vi "log_message.vi"(6 "timestamp":timestamp, 7 "context":string, 8 "error in (no error)":errorcluster, 9 "level":T1=400 items=["OFF"=0, "FATAL"=100, "ERROR"=200, "WARN"=300, "INFO"=400, "DEBUG"=500, "TRACE"=600, "ALL"=65535], 10 "message":string, 11 "Log Service in":refnum<class "Log Service.lvclass">) -> (0 "error out":errorcluster, 3 "Log Service out":refnum<class "Log Service.lvclass">)   [LabVIEW 2019, in "LVCOOOP.lvlib" / "Support API.lvlib" / "Log Service.lvclass"]
uses:
  Log Service.lvclass
  public/level.ctl
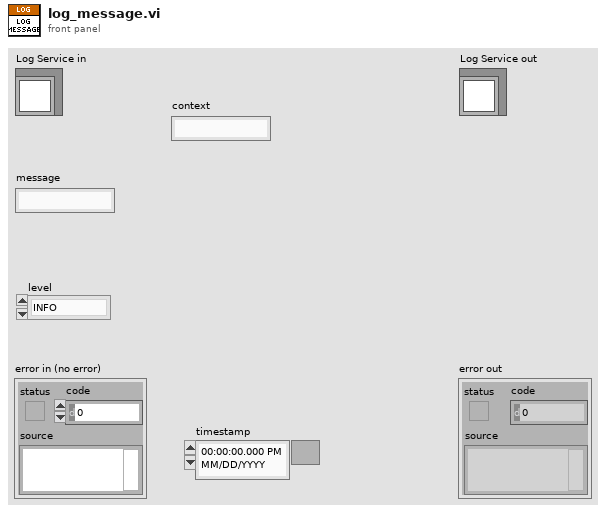
[diagram p1: front panel]
types:
  T1 = typedef "LVCOOOP.lvlib/Support API.lvlib/Log Service.lvclass/level.ctl" = u16
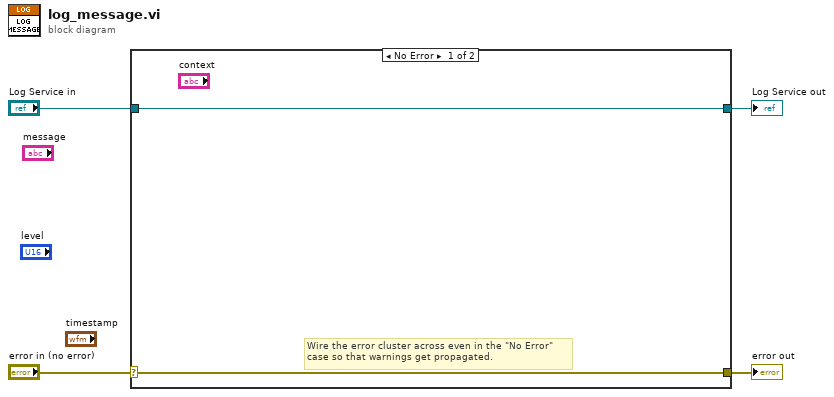
[diagram p0: block diagram]
diagram:
  n1 = case shown="No Error" "error in (no error)" {
    selector: "error in (no error)" -> [w5 w8]
    tunnel: [w5 w8] -> w3
    tunnel: [w6 w7] -> w1
    tunnel: "Log Service in" -> [w6 w7]
    frame No Error {
      # "Wire the error cluster across even in the \"No Error\"\ncase so that warnings get propagated."
    }
    frame Error {
    }
  }
  "error out" <- w3
  "Log Service out" <- w1
